vi "Simple Get Multiple Files.vi"(0 "host uri":string, 1 "username":string, 2 "password":string, 5 "file specifications":T1(array[cluster]), 11 "error in (no error)":errorcluster) -> (15 "error out":errorcluster)   [LabVIEW 2020, in "NI_WebDAV.lvlib"]
doc: "Returns a file or multiple files or the raw binary contents of a file or multiple files from a remote WebDAV server or target. You must manually select the polymorphic instance you want to use."
uses:
  <vilib>/WebDAVClient/NI_WebDAV.lvlib
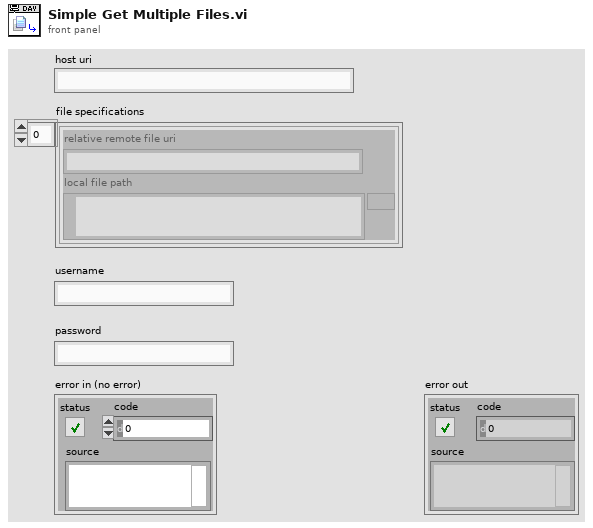
[diagram p1: front panel]
types:
  T1 = cluster{"relative remote file uri":string, "local file path":path}[]
  T2 = typedef "NI_WebDAV.lvlib/SessionHandle.ctl" = refnum<k1>
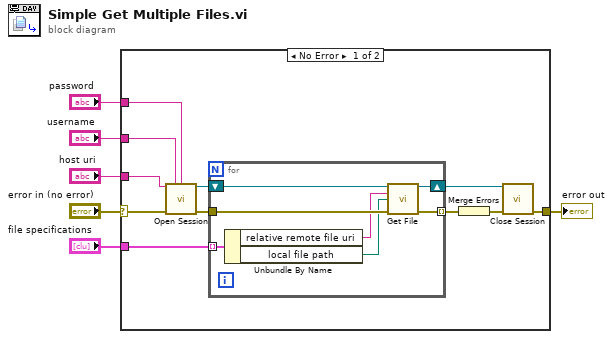
[diagram p0: block diagram]
diagram:
  n1 = case shown="No Error" "error in (no error)" {
    selector: "error in (no error)" -> [w17 w25]
    tunnel: "host uri" -> [w16 _]
    tunnel: "username" -> [w15 _]
    tunnel: "password" -> [w14 _]
    tunnel: "file specifications" -> [w11 _]
    tunnel: [w8 w25] -> w1
    frame No Error {
      n2 = call <vilib>:"Open Session.vi"("host uri prefix"=w16, "username"=w15, "password"=w14, "error in (no error)"=w17) -> ("session handle out"=w12:T2, "error out"=w13:errorcluster)  [unwired: 10 in]
      n3 = for {
        tunnel: w11 -> [w24] mode=indexing
        tunnel: w13 -> [w23]
        shift-right: [w19] -> w9
        shift-left: w12 -> [w22]
        tunnel: [w18] -> w7 mode=indexing
        n4 = Unbundle By Name(w24) -> ("relative remote file uri"=w21:string, "local file path"=w20:path)
        n5 = call <vilib>:"Get File.vi"("session handle"=w22, "relative uri"=w21, "local file path"=w20, "error in (no error)"=w23) -> ("session handle out"=w19:T2, "error out"=w18:errorcluster)  [unwired: 9 in, 1 out]
      }
      n6 = Merge Errors(w7) -> (w10:errorcluster)
      n7 = call <vilib>:"Close Session.vi"("session handle"=w9, "error in (no error)"=w10) -> ("error out"=w8:errorcluster)  [unwired: 13 in]
    }
    frame Error {
    }
  }
  "error out" <- w1
